vi "XY Graph Change X Axis Origin.vi"(6 "Shift (F)":bool, 8 "Error In":errorcluster, 9 "New X Origin (0)":dbl, 11 "Plot in":cluster{"X Array":dbl[], "Y Array":dbl[]}) -> (0 "Error Out":errorcluster, 1 "Shift":dbl, 3 "Plot out":cluster{"X Array":dbl[], "Y Array":dbl[]})   [LabVIEW 2021, in "XY Graph Add-Ons.lvlib"]
doc: "Conditionally shifts the plot's X axis such that the first value is equal to the <B>New X Origin</B> parameter.\n\nReturns the resulting <B>Shift</B> parameter (New X Origin - Old X Origin)."
uses:
  XY Graph Add-Ons.lvlib
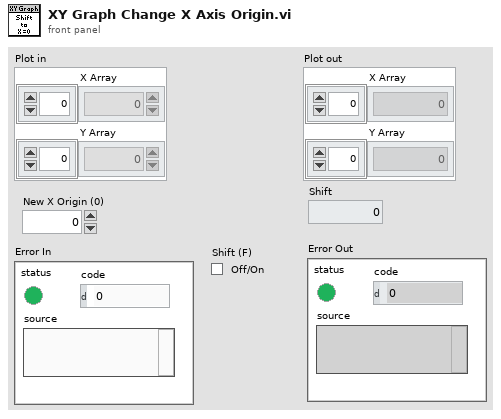
[diagram p1: front panel]
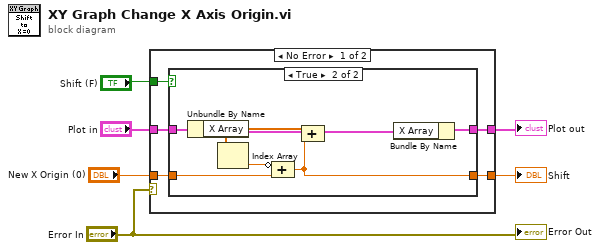
[diagram p0: block diagram]
diagram:
  n1 = case shown="No Error" "Error In" {
    tunnel: "Shift (F)" -> [w11 _]
    tunnel: "Plot in" -> [w10 w20]
    tunnel: [w9 w20] -> w4
    tunnel: [w8 _] -> w3
    tunnel: "New X Origin (0)" -> [w7 _]
    frame No Error {
      n2 = case shown="True" w11 {
        tunnel: w10 -> [w12 w19]
        tunnel: [w12 w18] -> w9
        tunnel: [_ w13] -> w8
        tunnel: w7 -> [_ w14]
        frame False {
        }
        frame True {
          n3 = Unbundle By Name(w19) -> ("X Array"=w17:dbl[])
          n4 = Index Array(array=w17) -> (element=w15:dbl)  [unwired: 1 in]
          n5 = Compound Arithmetic op=ADD(invert w15, w14) -> (w13:dbl)
          n6 = Compound Arithmetic op=ADD(w17, w13) -> (w16:dbl[])
          n7 = Bundle By Name(cluster=w19, "X Array"=w16) -> (w18:cluster{"X Array":dbl[], "Y Array":dbl[]})
        }
      }
    }
    frame Error {
    }
  }
  "Plot out" <- w4
  "Shift" <- w3
  "Error Out" <- "Error In"
